vi "BuildContentXML.vi"() -> ()   [LabVIEW 2014]
panel:
  out "Equal?":bool
  out "Calc'd Content.XML":string
  out "Content.XML":string
  in  "SpreadsheetData":T1(array[cluster])
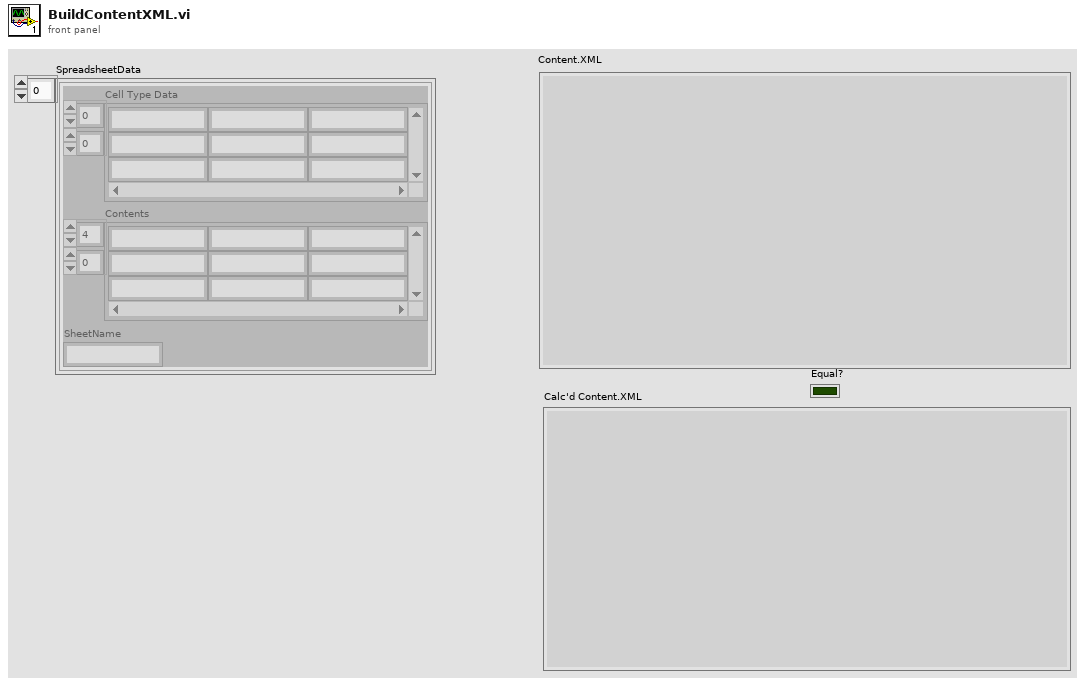
[diagram p1: front panel]
types:
  T1 = cluster{"Cell Type Data":string[][], "Contents":string[][], "SheetName":string}[]
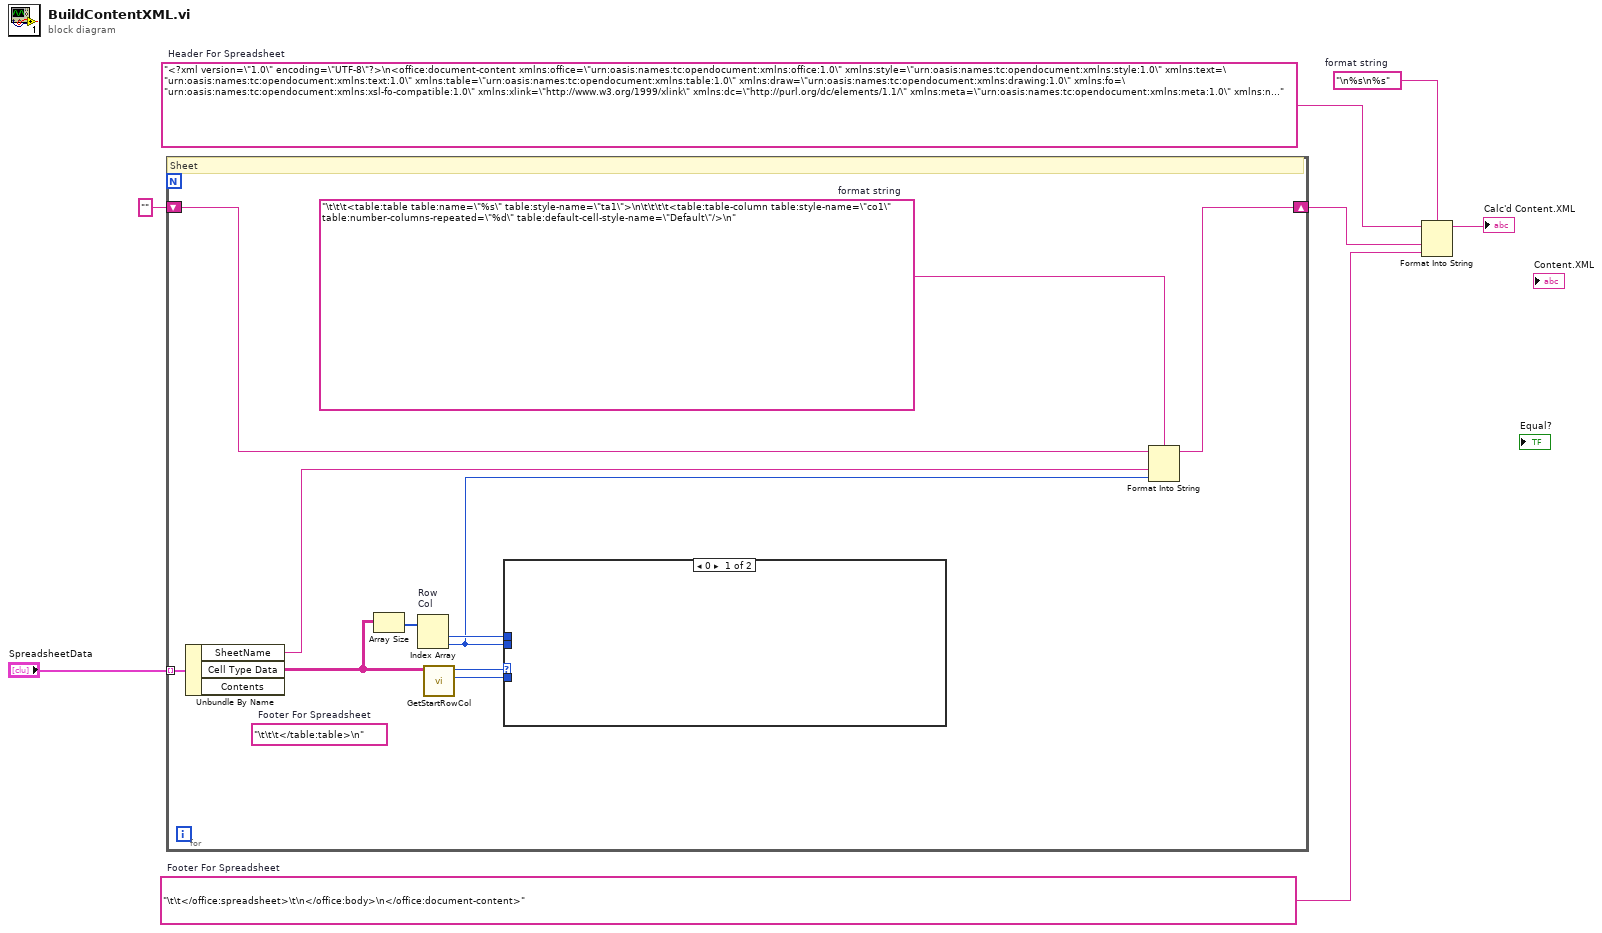
[diagram p0: block diagram]
diagram:
  w2 = "\t\t</office:spreadsheet>\t\n</office:body>\n</office:document-content>"  # Footer For Spreadsheet
  w5 = "\n%s\n%s"  # format string
  w6 = "<?xml version=\"1.0\" encoding=\"UTF-8\"?>\n<office:document-content xmlns:office=\"urn:oasis:names:tc:opendocument:xmlns:office:1.0\" xmlns:style=\"urn:oasis:names:tc:opendocument:xmlns:style:1.0\" xmlns:text=\"urn:oasis:names:tc:opendocument:xmlns:text:1.0\" xmlns:table=\"urn:oasis:names:tc:opendocument:xmlns:table:1.0\" xmlns:draw=\"urn:oasis:names:tc:opendocument:xmlns:drawing:1.0\" xmlns:fo=\"urn:oasis:names:tc:opendocument:xmlns:xsl-fo-compatible:1.0\" xmlns:xlink=\"http://www.w3.org/1999/xlink\" xmlns:dc=\"http://purl.org/dc/elements/1.1/\" xmlns:meta=\"urn:oasis:names:tc:opendocument:xmlns:meta:1.0\" xmlns:number=\"urn:oasis:names:tc:opendocument:xmlns:datastyle:1.0\" xmlns:presentation=\"urn:oasis:names:tc:opendocument:xmlns:presentation:1.0\" xmlns:svg=\"urn:oasis:names:tc:opendocument:xmlns:svg-compatible:1.0\" xmlns:chart=\"urn:oasis:names:tc:opendocument:xmlns:chart:1.0\" xmlns:dr3d=\"urn:oasis:names:tc:opendocument:xmlns:dr3d:1.0\" xmlns:math=\"http://www.w3.org/1998/Math/MathML\" xmlns:form=\"urn:oasis:names:tc:opendocument:xmlns:form:1.0\" xmlns:script=\"urn:oasis:names:tc:opendocument:xmlns:script:1.0\" xmlns:ooo=\"http://openoffice.org/2004/office\" xmlns:ooow=\"http://openoffice.org/2004/writer\" xmlns:oooc=\"http://openoffice.org/2004/calc\" xmlns:dom=\"http://www.w3.org/2001/xml-events\" xmlns:xforms=\"http://www.w3.org/2002/xforms\" xmlns:xsd=\"http://www.w3.org/2001/XMLSchema\" xmlns:xsi=\"http://www.w3.org/2001/XMLSchema-instance\" xmlns:rpt=\"http://openoffice.org/2005/report\" xmlns:of=\"urn:oasis:names:tc:opendocument:xmlns:of:1.2\" xmlns:xhtml=\"http://www.w3.org/1999/xhtml\" xmlns:grddl=\"http://www.w3.org/2003/g/data-view#\" xmlns:tableooo=\"http://openoffice.org/2009/table\" xmlns:drawooo=\"http://openoffice.org/2010/draw\" xmlns:calcext=\"urn:org:documentfoundation:names:experimental:calc:xmlns:calcext:1.0\" xmlns:loext=\"urn:org:documentfoundation:names:experimental:office:xmlns:loext:1.0\" xmlns:field=\"urn:openoffice:names:experimental:ooo-ms-interop:xmlns:field:1.0\" xmlns:formx=\"urn:openoffice:names:experimental:ooxml-odf-interop:xmlns:form:1.0\" xmlns:css3t=\"http://www.w3.org/TR/css3-text/\" office:version=\"1.2\">\n\t<office:scripts/>\n\t<office:font-face-decls>\n\t\t<style:font-face style:name=\"Liberation Sans\" svg:font-family=\"&apos;Liberation Sans&apos;\" style:font-family-generic=\"swiss\" style:font-pitch=\"variable\"/>\n\t\t<style:font-face style:name=\"Mangal\" svg:font-family=\"Mangal\" style:font-family-generic=\"system\" style:font-pitch=\"variable\"/>\n\t\t<style:font-face style:name=\"Microsoft YaHei\" svg:font-family=\"&apos;Microsoft YaHei&apos;\" style:font-family-generic=\"system\" style:font-pitch=\"variable\"/>\n\t\t<style:font-face style:name=\"Segoe UI\" svg:font-family=\"&apos;Segoe UI&apos;\" style:font-family-generic=\"system\" style:font-pitch=\"variable\"/>\n\t\t<style:font-face style:name=\"Tahoma\" svg:font-family=\"Tahoma\" style:font-family-generic=\"system\" style:font-pitch=\"variable\"/>\n\t</office:font-face-decls>\n\t<office:automatic-styles>\n\t\t<style:style style:name=\"co1\" style:family=\"table-column\">\n\t\t\t<style:table-column-properties fo:break-before=\"auto\" style:column-width=\"22.58mm\"/>\n\t\t</style:style>\n\t\t<style:style style:name=\"ro1\" style:family=\"table-row\">\n\t\t\t<style:table-row-properties style:row-height=\"4.52mm\" fo:break-before=\"auto\" style:use-optimal-row-height=\"true\"/>\n\t\t</style:style>\n\t\t<style:style style:name=\"ta1\" style:family=\"table\" style:master-page-name=\"Default\">\n\t\t\t<style:table-properties table:display=\"true\" style:writing-mode=\"lr-tb\"/>\n\t\t</style:style>\n\t</office:automatic-styles>\n\t<office:body>\n\t\t<office:spreadsheet>"  # Header For Spreadsheet
  n1 = for {
    tunnel: "SpreadsheetData" -> [w18] mode=indexing
    shift-right: [w12] -> w3
    shift-left: "" -> [w17]
    (unwired) "\t\t\t</table:table>\n"  # Footer For Spreadsheet
    w16 = "\t\t\t<table:table table:name=\"%s\" table:style-name=\"ta1\">\n\t\t\t\t<table:table-column table:style-name=\"co1\" table:number-columns-repeated=\"%d\" table:default-cell-style-name=\"Default\"/>\n"  # format string
    # "Sheet"
    n2 = Unbundle By Name(w18) -> ("SheetName"=w15:string, "Cell Type Data"=w14:string[][])  [unwired: 1 out]
    n3 = Array Size(array=w14) -> (size(s)=w13:i32[])
    n4 = Index Array "Row\nCol"(array=w13) -> (element #1=w10:i32, element #2=w8:i32)  [unwired: 2 in]
    n5 = call "GetStartRowCol.vi"("Cell Type Data"=w14) -> ("#Cols Empty"=w9:i32, "#Rows Empty"=w11:i32)  [unwired: 9 in]
    n6 = case shown="0" w11 {
      tunnel: w10 -> [_ _]
      tunnel: w8 -> [_ _]
      tunnel: w9 -> [_ _]
      frame 0 {
      }
      frame 1, Default {
      }
    }
    n7 = Format Into String(format string=w16, initial string=w17, w15, w8) -> (resulting string=w12:string)  [unwired: 1 in, 1 out]
  }
  n8 = Format Into String(format string=w5, initial string=w6, w3, w2) -> (resulting string=→"Calc'd Content.XML":string)  [unwired: 1 in, 1 out]
